vi "Module Template.vi"   [LabVIEW 2020, in "Publisher Subscriber.lvlib"]
uses:
  Publisher Subscriber.lvlib
  Controls/node refnum.ctl
  ae88ff53-e2b6-4b5a-85aa-5b466751ef77.vi
types:
  T1 = typedef "Publisher Subscriber.lvlib/node refnum.ctl" = refnum<k1>
  T2 = cluster{"Node Ref":T1, "Message":string, "Tout":i32}
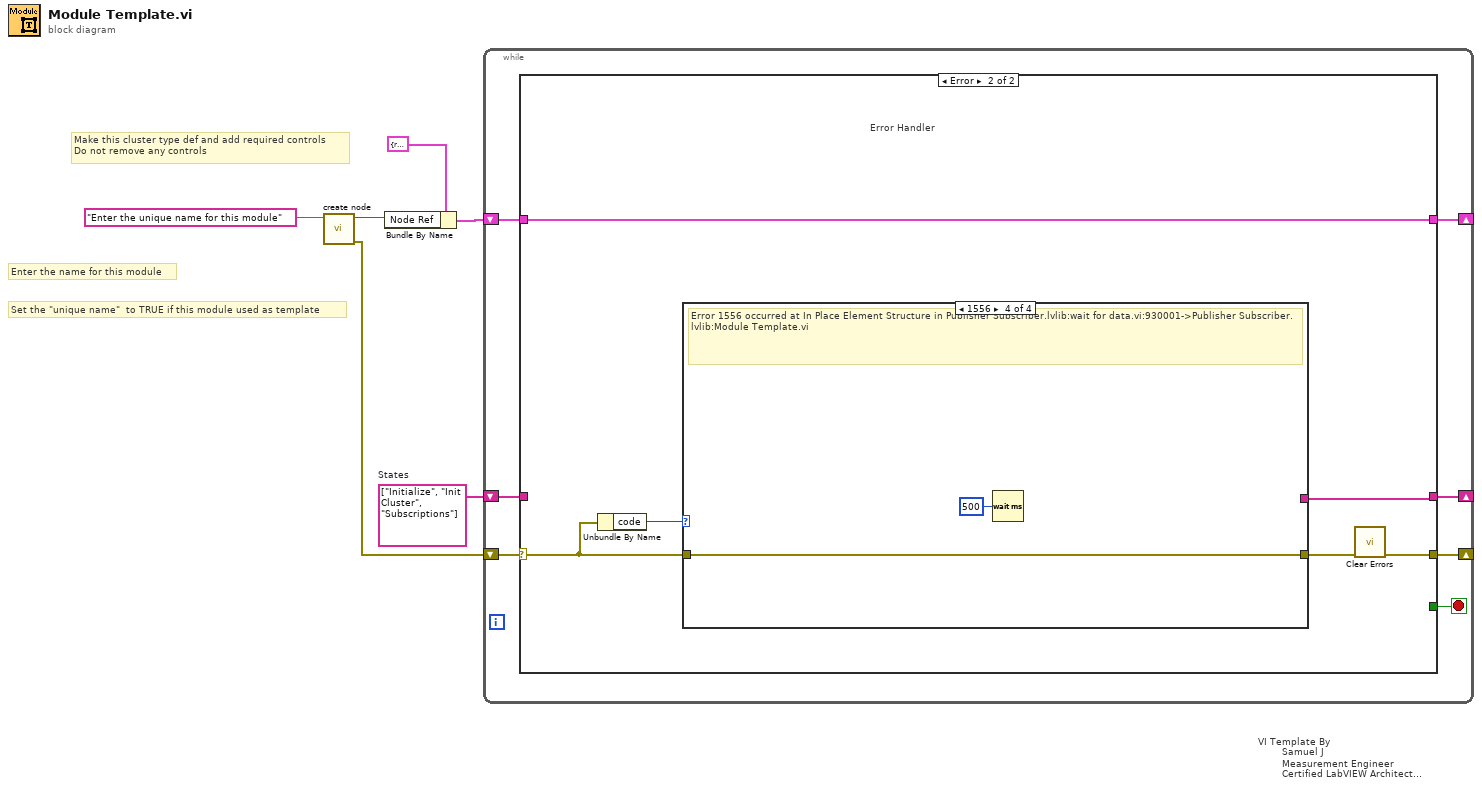
[diagram p0: block diagram]
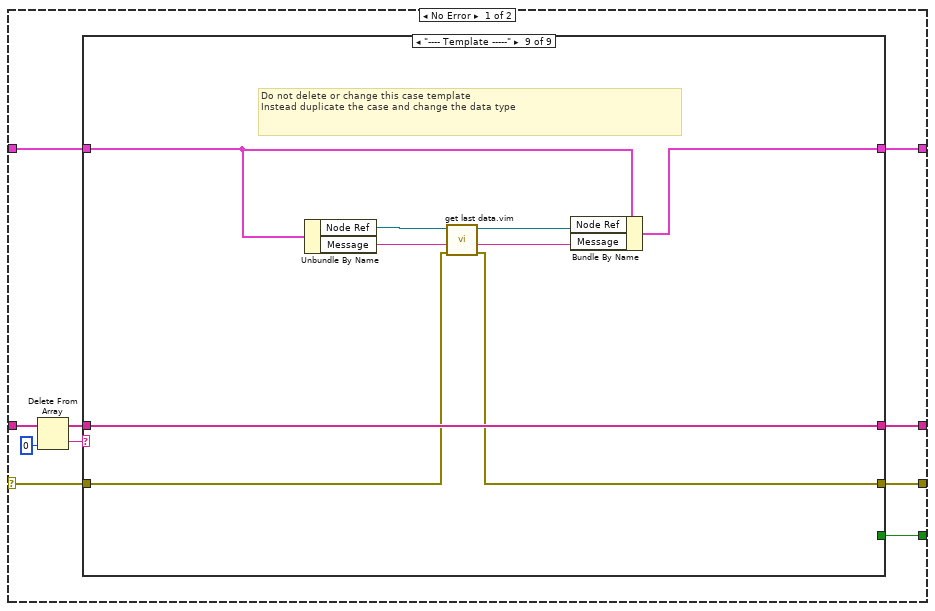
[diagram p2: hidden frame]
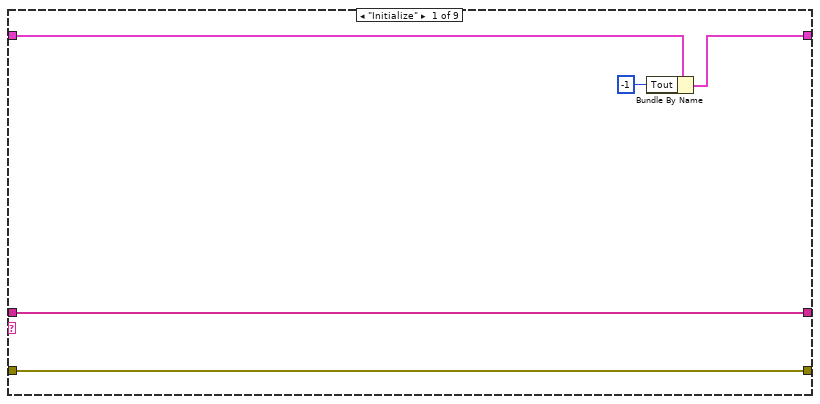
[diagram p3: hidden frame]
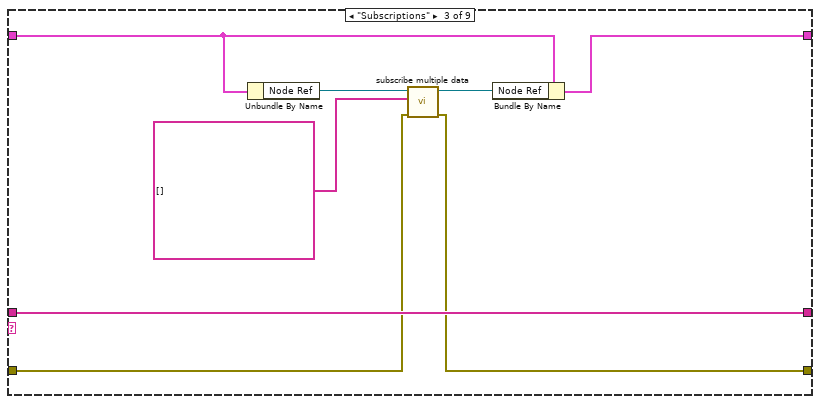
[diagram p5: hidden frame]
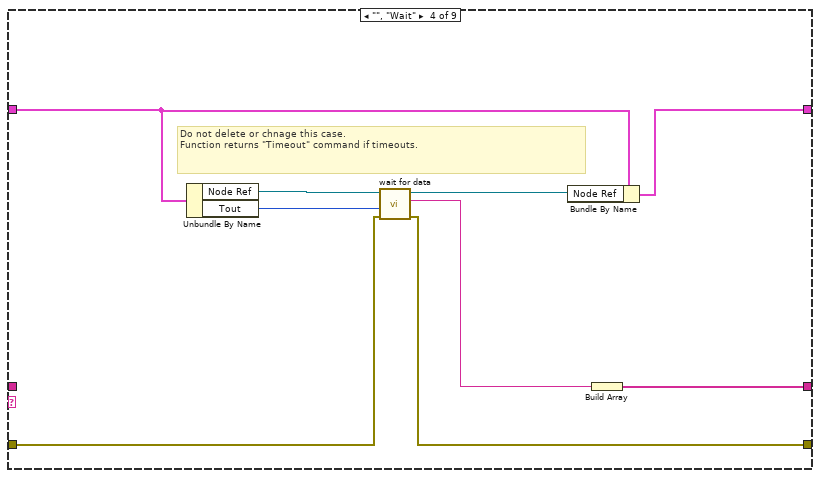
[diagram p6: hidden frame]
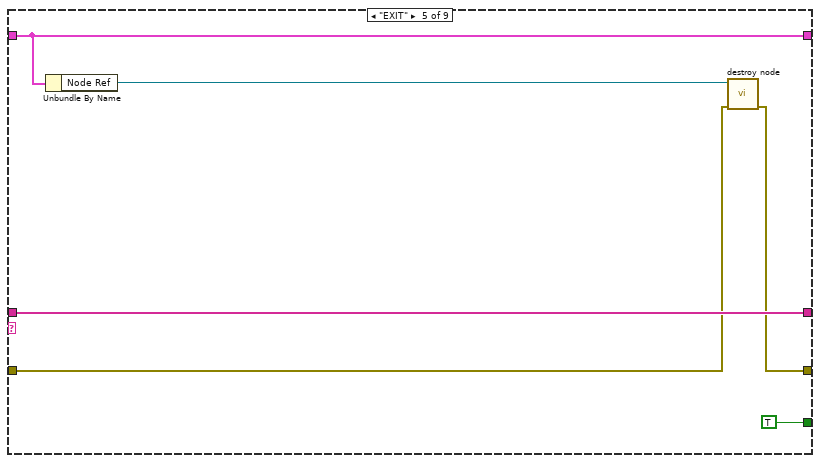
[diagram p7: hidden frame]
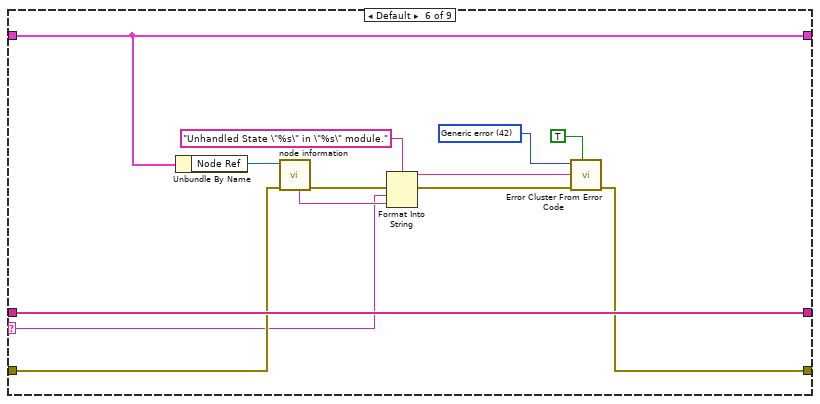
[diagram p8: hidden frame]
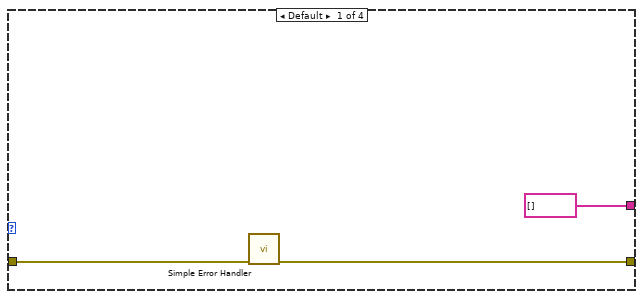
[diagram p11: hidden frame]
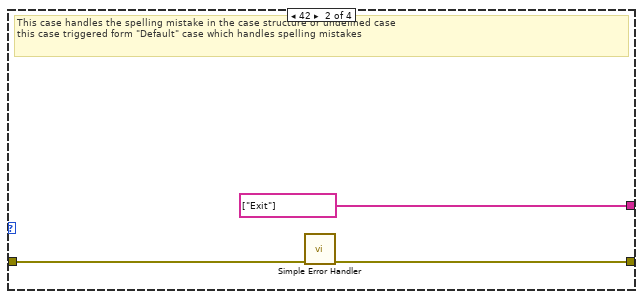
[diagram p12: hidden frame]
diagram:
  w6 = string[] ["Initialize", "Init Cluster", "Subscriptions"]  # States
  # "Set the \"unique name\"  to TRUE if this module used as template"
  # "Enter the name for this module"
  # "Make this cluster type def and add required controls\nDo not remove any controls"
  n1 = call "create node.vi"("node name"="Enter the unique name for this module" ("Subscriber name")) -> ("error out"=w1:errorcluster, "node ref out"=w3:T1)  [unwired: 9 in]
  n2 = Bundle By Name(cluster=T2 {"Node Ref"=refnum, "Message"="", "Tout"=-1} ("Cluster"), "Node Ref"=w3) -> (w4:T2)
  n3 = while "VI Template By\n        Samuel J\n        Measurement Engineer\n        Certified LabVIEW Architect\n        Vestas Technology R&D Chennai" {
    shift-right: [w9] -> _
    shift-left: w6 -> [w13]
    shift-right: [w10] -> _
    shift-left: w1 -> [w12]
    shift-right: [w8] -> _
    shift-left: w4 -> [w11]
    stop <- w7 stop-if-true
    n4 = case shown="Error" w12 {
      selector: w12 -> [w18 w86]
      tunnel: w13 -> [w22 _]
      tunnel: w11 -> [w19 w88]
      tunnel: [w17 w84] -> w10
      tunnel: [w16 w83] -> w9
      tunnel: [w15 w88] -> w8
      tunnel: [w14 _] -> w7
      frame No Error {
        n5 = Delete From Array(array=w22, index=0) -> (deleted portion=w21:string, array with subset deleted=w20:string[])  [unwired: 1 in]
        n6 = case shown="\"---- Template -----\"" w21 {
          selector: w21 -> [_ _ _ _ _ w56 _ _ _]
          tunnel: w20 -> [w28 w30 w39 _ w54 w67 w69 w72 w82]
          tunnel: w19 -> [w26 w29 w36 w47 w51 w58 w68 w71 w79]
          tunnel: w18 -> [w24 w31 w33 w45 w49 w57 w70 w73 w76]
          tunnel: [w24 w31 w34 w43 w50 w55 w70 w73 w77] -> w17
          tunnel: [w28 w30 w39 w41 w54 w67 w69 w72 w82] -> w16
          tunnel: [w27 w29 w37 w40 w51 w58 w68 w71 w80] -> w15
          tunnel: [_ _ _ _ TRUE ("Exit") _ _ _ _] -> w14
          frame "Initialize" {
            n7 = Bundle By Name(cluster=w26, "Tout"=-1) -> (w27:T2)
          }
          frame "Init Cluster" {
          }
          frame "Subscriptions" {
            n8 = Unbundle By Name(w36) -> ("Node Ref"=w38:T1)
            n9 = call "subscribe multiple data.vi"("error in"=w33, "subriscription list[]"=string[] [], "refnum in"=w38) -> ("error out"=w34:errorcluster, "refnum out"=w35:T1)  [unwired: 7 in]
            n10 = Bundle By Name(cluster=w36, "Node Ref"=w35) -> (w37:T2)
          }
          frame "", "Wait" {
            # "Do not delete or chnage this case.\nFunction returns \"Timeout\" command if timeouts."
            n11 = Unbundle By Name(w47) -> ("Node Ref"=w48:T1, "Tout"=w46:i32)
            n12 = call "wait for data.vi"("error in"=w45, "timeout in ms (-1)"=w46, "refnum in"=w48) -> ("error out"=w43:errorcluster, "command"=w42:string, "refnum out"=w44:T1)  [unwired: 5 in, 1 out]
            n13 = Bundle By Name(cluster=w47, "Node Ref"=w44) -> (w40:T2)
            n14 = Build Array(w42) -> (w41:string[])
          }
          frame "EXIT" {
            n15 = Unbundle By Name(w51) -> ("Node Ref"=w52:T1)
            n16 = call "destroy node.vi"("error in"=w49, "refnum in"=w52) -> ("error out"=w50:errorcluster)  [unwired: 8 in, 1 out]
          }
          frame Default {
            w63 = 42 items=["No error", "Argument error", "Memory is full", "Out of zone", "End of file", "File already open", "Generic file I/O error", "File not found", "File permission error", "Disk is full", "Duplicate path", "Too many files open", "System feature not enabled", "Resource file not found", "Cannot add resource", "Resource not found", "Image not found", "Image memory error", "Pen does not exist", "Config type invalid", "Config token not found", "Config parse error", "Config memory error", "Bad external code format", "Bad external code offset", "External code not present", "Null window", "Destroy window error", "Null menu", "Print aborted", "Bad print record", "Print driver error", "Windows error during printing", "Memory error during printing", "Print dialog error", "Generic print error", "Invalid device refnum", "Device not found", "Device parameter error", "Device unit error", "Cannot open device", "Device call aborted", "Generic error", "Cancelled by user", "Object ID too low", "Object ID too high", "Object not in heap", "Unknown heap", "Unknown object (invalid DefProc)", "Unknown object (DefProc not in table)", "Message out of range", "Invalid (null) method", "Unknown message", "Manager call not supported", "Bad address", "Network operation in progress", "Network operation timed out", "Connection is busy", "Network attribute not supported", "Network error", "Address in use", "System out of memory", "Connection aborted", "Connection refused", "Not connected", "Already connected", "Connection closed", "Initialization error (interapplication manager)", "Bad occurrence", "Wait on unbound occurrence handler", "Occurrence queue overflow", "Datalog type conflict", "Unused", "Unrecognized type (interapplication manager)", "Memory corrupt", "Failed to make temporary DLL", "Old CIN version", "Drag socket not found", "Failed to load drop-object", "Failed to register OLE object", "Failed to release OLE object", "Format specifier type mismatch", "Unknown format specifier", "Too few format specifiers", "Too many format specifiers", "Scan failed", "Newer CIN version", "Error converting to variant", "Runtime menu error", "Password tampered", "Variant attribute not found", "Incompatible variant data type", "Event data is not available", "Event Store is not present", "Occurrence is not found", "Event Queue is not created", "Event info is not available", "Refnum passed is NULL", "Error retrieving Class GUID", "Error retrieving CoClass GUID", "Error retrieving TypeLib GUID.", "Bad built application magic bytes.", "Specific driver is different from the specific driver associated with the Logical Name.", "There is no session opened to the class driver.", "Max Error", "MAX - Error with config objects", "MAX - Error loading configuration", "MAX - Group not supported"]
            n17 = Unbundle By Name(w58) -> ("Node Ref"=w61:T1)
            n18 = call "node information.vi"("error in"=w57, "refnum in"=w61) -> ("error out"=w59:errorcluster, "this node name"=w60:string)  [unwired: 4 in, 4 out]
            n19 = Format Into String(format string="Unhandled State \"%s\" in \"%s\" module." ("message"), error in=w59, w56, w60) -> (resulting string=w64:string, error out=w65:errorcluster)  [unwired: 1 in]
            n20 = call <vilib>:"Error Cluster From Error Code.vi"("show call chain? (False)"=TRUE, "error in (no error)"=w65, "error message (\"\")"=w64, "error code (0)"=w63) -> ("error out"=w55:errorcluster)  [unwired: 5 out]
          }
          frame "Timeout" {
            # "Do not delete this case, Put your timeout code here"
          }
          frame "======== DATA =========" {
          }
          frame "---- Template -----" {
            # "Do not delete or change this case template \nInstead duplicate the case and change the data type"
            n21 = Unbundle By Name(w79) -> ("Node Ref"=w81:T1, "Message"=w75:string)
            n22 = call "get last data.vim"("error in"=w76, "data type"=w75, "refnum in"=w81) -> ("error out"=w77:errorcluster, "data out"=w74:string, "refnum out"=w78:T1)  [unwired: 5 in, 1 out]
            n23 = Bundle By Name(cluster=w79, "Node Ref"=w78, "Message"=w74) -> (w80:T2)
          }
        }
      }
      frame Error {
        # "Error Handler"
        n24 = Unbundle By Name(w86) -> ("code"=w87:i32)
        n25 = case shown="1556" w87 {
          tunnel: w86 -> [w91 w92 w95 w96]
          tunnel: [w90 w93 w95 w96] -> w85
          tunnel: [string[] [] ("States") string[] ["Exit"] ("States") _ _] -> w83
          frame Default {
            n26 = call <vilib>:"Simple Error Handler.vi"("error in (no error)"=w91) -> ("error out"=w90:errorcluster)  [unwired: 1 in, 7 out]
          }
          frame 42 {
            # "This case handles the spelling mistake in the case structure or undefined case\nthis case triggered form \"Default\" case which handles spelling mistakes"
            n27 = call <vilib>:"Simple Error Handler.vi"("error in (no error)"=w92) -> ("error out"=w93:errorcluster)  [unwired: 1 in, 7 out]
          }
          frame 5701 {
            # "Error 5701 occurred at Node with the name \"Enter the unique name here\"\nalready exists. Provide unique name for the node."
          }
          frame 1556 {
            # "Error 1556 occurred at In Place Element Structure in Publisher Subscriber.lvlib:wait for data.vi:930001->Publisher Subscriber.lvlib:Module Template.vi"
            n28 = Wait (ms)(milliseconds to wait=u32 500) -> ()  [unwired: 1 out]
          }
        }
        n29 = call <vilib>:"Clear Errors.vi"("error in (no error)"=w85) -> ("error out"=w84:errorcluster)  [unwired: 1 in, 5 out]
      }
    }
  }
